vi "send.status.vi"(6 "iteration":i32, 8 "error in (no error)":errorcluster, 11 "ComicVine_manager in":refnum<class "CV_downloader.lvclass">) -> (0 "error out":errorcluster, 3 "ComicVine_manager out":refnum<class "CV_downloader.lvclass">)   [LabVIEW 2024, in "CV_downloader.lvclass"]
uses:
  CV_downloader.lvclass
  CV_downloader.lvclass/CV_downloader.ctl
  status--cluster.ctl
  9bd0a203-ee3b-45b2-a7a7-44ce231499cd.vi
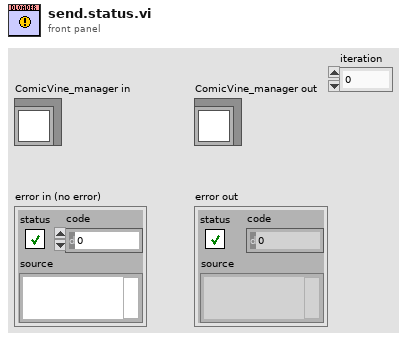
[diagram p1: front panel]
types:
  T1 = typedef "CV_downloader.lvclass/status--cluster.ctl" = cluster{"files in queue":i32, "in jail?":bool, "current state":string, "time left (s)":dbl, "iteration":i32, "error status":errorcluster, "log file":path, "Approx Completion":timestamp, "updated item":string}
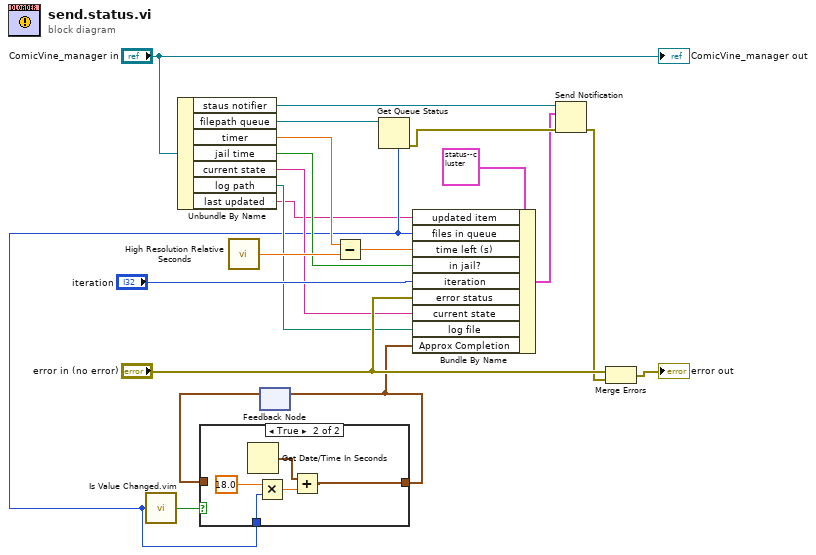
[diagram p0: block diagram]
diagram:
  n1 = Unbundle By Name("ComicVine_manager in") -> ("staus notifier"=w20:refnum<notifier>, "filepath queue"=w18:refnum<queue>, "timer"=w16:dbl, "jail time"=w13:bool, "current state"=w7:string, "log path"=w6:path, "last updated"=w1:string)
  n2 = call <vilib>:"High Resolution Relative Seconds.vi"() -> ("relative seconds"=w15:dbl)
  n3 = feedback #1() -> (w4:timestamp)  [unwired: 1 in]
  n4 = Subtract(x=w16, y=w15) -> (x-y=w14:dbl)
  n5 = Get Queue Status(queue=w18) -> (error out=w17:errorcluster, # elements in queue=w3:i32)  [unwired: 2 in, 6 out]
  n6 = call "Is Value Changed.vim"("value"=w3) -> ("changed or first call?"=w5:bool)
  n7 = case shown="True" w5 {
    tunnel: [w22 w25] -> w2
    tunnel: w4 -> [w22 _]
    tunnel: w3 -> [_ w23]
    frame False {
    }
    frame True {
      n8 = Get Date/Time In Seconds() -> (seconds since 1Jan1904=w26:timestamp)
      n9 = Multiply(x=18.0, y=w23) -> (x*y=w27:dbl)
      n10 = Add(x=w26, y=w27) -> (x+y=w25:timestamp)
    }
  }
  n11 = feedback-in #1(w2) -> ()
  n12 = Bundle By Name(cluster=T1 {"files in queue"=0, "in jail?"=FALSE, "current state"="", "time left (s)"=0.0, "iteration"=0, "error status"={"status"=FALSE, "code"=0, "source"=""}, "log file"=path "", "Approx Completion"=timestamp(0 s since 1904-01-01), "updated item"=""} ("status"), "updated item"=w1, "files in queue"=w3, "time left (s)"=w14, "in jail?"=w13, "iteration"="iteration", "error status"="error in (no error)", "current state"=w7, "log file"=w6, "Approx Completion"=w2) -> (w12:T1)
  n13 = Send Notification(notification=w12, notifier=w20, error in (no error)=w17) -> (error out=w9:errorcluster)  [unwired: 1 out]
  n14 = Merge Errors("error in (no error)", w9) -> (→"error out":errorcluster)
  "ComicVine_manager out" <- "ComicVine_manager in"
